vi "Cycle.vi"(6 "Measure Cycles":bool, 8 "error in (no error)":errorcluster, 9 "Cycles":i32, 10 "Cycle Write Outfile":path, 11 "IVI Refnum in":refnum<k15>) -> (0 "error out":errorcluster, 1 "currents (A)":dbl[](array[numeric]), 2 "resistances (ohm)":dbl[](array[numeric]), 3 "IVI Refnum out":refnum<k15>)   [LabVIEW 2018]
uses:
  Globals.vi
  <vilib>/Utility/file.llb/Write Delimited Spreadsheet (DBL).vi
panel:
  out "i":i32
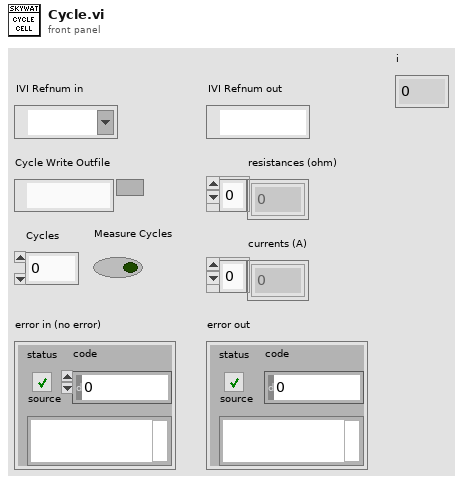
[diagram p1: front panel]
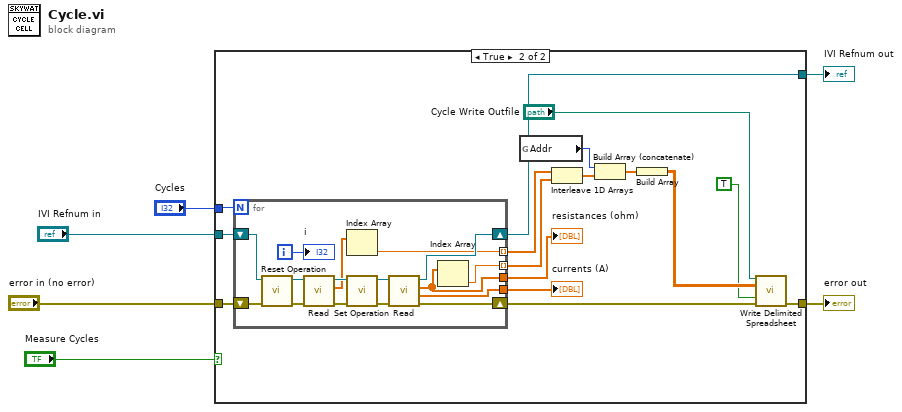
[diagram p0: block diagram]
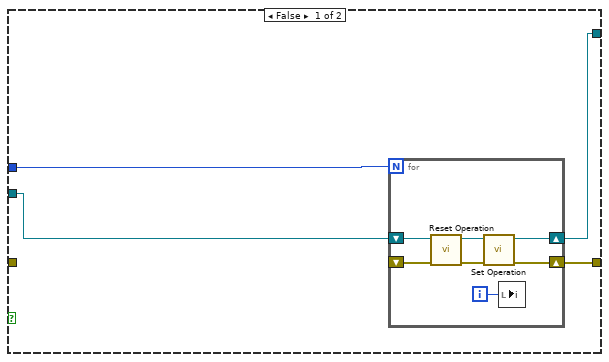
[diagram p2: hidden frame]
diagram:
  n1 = case shown="True" "Measure Cycles" {
    tunnel: [w9 w33] -> w6
    tunnel: "error in (no error)" -> [_ w21]
    tunnel: "IVI Refnum in" -> [w10 w20]
    tunnel: "Cycles" -> [w7 w19]
    tunnel: [w8 w18] -> w1
    frame False {
      n2 = for {
        N: w7 -> [_]
        shift-right: [w11] -> w8
        shift-left: w10 -> [w17]
        shift-right: [w13] -> w9
        shift-left: _ -> [w16]
        i -> [w15]
        n3 = call "Reset Operation.vi"("error in (no error)"=w16, "instrument handle"=w17) -> ("error out"=w14:errorcluster, "instrument handle out"=w12:refnum<k15>)  [unwired: 8 in]
        n4 = call "Set Operation.vi"("error in (no error)"=w14, "instrument handle"=w12) -> ("error out"=w13:errorcluster, "instrument handle out"=w11:refnum<k15>)  [unwired: 8 in]
        n5 = local write "i"(w15) -> ()
      }
    }
    frame True {
      n6 = for {
        N: w19 -> [_]
        shift-right: [w43] -> w18
        shift-left: w20 -> [w42]
        shift-right: [w40] -> w32
        shift-left: w21 -> [w41]
        tunnel: [w38] -> w22
        tunnel: [w39] -> w23
        tunnel: [w36] -> w25 mode=indexing
        tunnel: [w35] -> w26 mode=indexing
        i -> [w34]
        n7 = call "Reset Operation.vi"("error in (no error)"=w41, "instrument handle"=w42) -> ("error out"=w49:errorcluster, "instrument handle out"=w48:refnum<k15>)  [unwired: 8 in]
        n8 = call "Read.vi"("error in (no error)"=w49, "instrument handle"=w48) -> ("error out"=w47:errorcluster, "resistances (ohm)"=w37:dbl[], "instrument handle out"=w46:refnum<k15>)  [unwired: 6 in, 1 out]
        n9 = Index Array(array=w37) -> (element=w36:dbl)  [unwired: 1 in]
        n10 = call "Set Operation.vi"("error in (no error)"=w47, "instrument handle"=w46) -> ("error out"=w45:errorcluster, "instrument handle out"=w44:refnum<k15>)  [unwired: 8 in]
        n11 = call "Read.vi"("error in (no error)"=w45, "instrument handle"=w44) -> ("error out"=w40:errorcluster, "currents (A)"=w39:dbl[], "resistances (ohm)"=w38:dbl[], "instrument handle out"=w43:refnum<k15>)  [unwired: 6 in]
        n12 = Index Array(array=w38) -> (element=w35:dbl)  [unwired: 1 in]
        "i" <- w34
      }
      "currents (A)" <- w23
      "resistances (ohm)" <- w22
      n13 = global read "Globals.vi" "Addr"() -> (w28:i32)
      n14 = Interleave 1D Arrays(w25, w26) -> (w27:dbl[])
      n15 = Build Array (concatenate)(w28, w27) -> (w24:dbl[])
      n16 = Build Array(w24) -> (w31:dbl[][])
      n17 = call-poly <vilib>:"Write Delimited Spreadsheet.vi"("file path (dialog if empty)"="Cycle Write Outfile", "2D data"=w31, "append to file? (new file:F)"=TRUE, "error in (no error)"=w32) -> ("error out"=w33:errorcluster)  [unwired: 10 in, 1 out]
    }
  }
  "error out" <- w6
  "IVI Refnum out" <- w1
